vi "exit_node.vi"(5 "error in 3":errorcluster, 7 "task/channels in 3":refnum<k21>, 8 "error in 2":errorcluster, 9 "task/channels in 2":refnum<k21>, 10 "error in":errorcluster, 11 "task/channels in":refnum<k21>) -> ()   [LabVIEW 2014]
panel:
  # "Stop Node:\n\nConcatenates all Errors and Outputs"
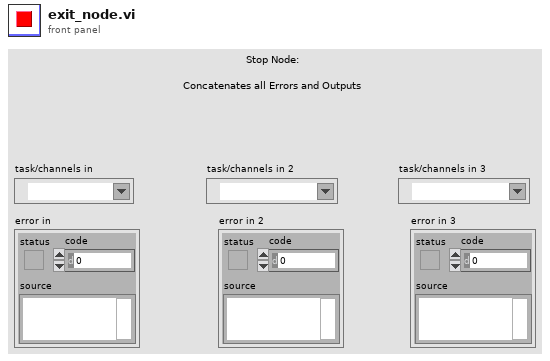
[diagram p1: front panel]
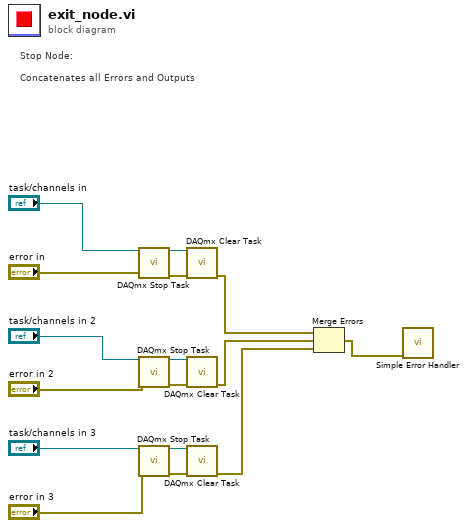
[diagram p0: block diagram]
diagram:
  # "Stop Node:\n\nConcatenates all Errors and Outputs"
  n1 = call <vilib>:"DAQmx Stop Task.vi"("task/channels in"="task/channels in", "error in"="error in") -> ("task out"=w16:refnum<k21>, "error out"=w15:errorcluster)  [unwired: 12 in]
  n2 = call <vilib>:"DAQmx Stop Task.vi"("task/channels in"="task/channels in 2", "error in"="error in 2") -> ("task out"=w10:refnum<k21>, "error out"=w11:errorcluster)  [unwired: 12 in]
  n3 = call <vilib>:"DAQmx Stop Task.vi"("task/channels in"="task/channels in 3", "error in"="error in 3") -> ("task out"=w9:refnum<k21>, "error out"=w8:errorcluster)  [unwired: 12 in]
  n4 = call <vilib>:"DAQmx Clear Task.vi"("task in"=w16, "error in"=w15) -> ("error out"=w14:errorcluster)  [unwired: 13 in]
  n5 = call <vilib>:"DAQmx Clear Task.vi"("task in"=w10, "error in"=w11) -> ("error out"=w13:errorcluster)  [unwired: 13 in]
  n6 = call <vilib>:"DAQmx Clear Task.vi"("task in"=w9, "error in"=w8) -> ("error out"=w12:errorcluster)  [unwired: 13 in]
  n7 = Merge Errors(w14, w13, w12) -> (w7:errorcluster)
  n8 = call <vilib>:"Simple Error Handler.vi"("error in (no error)"=w7) -> ()  [unwired: 4 in, 5 out]
